vi "CAP1208 Example.vi"() -> ()   [LabVIEW 2020]
uses:
  <vilib>/MakerHub/LINX/Public/Utilities/Open Local.vi
  LINX I2C/LINX I2C.lvclass
  <vilib>/MakerHub/LINX/LMH-LINX.lvlib
  CAP1208/CAP1208.lvclass
panel:
  out "Sensor Input (CS1-CS8)":bool[](array[boolean])
  out "error out":errorcluster
  in  "Stop":bool
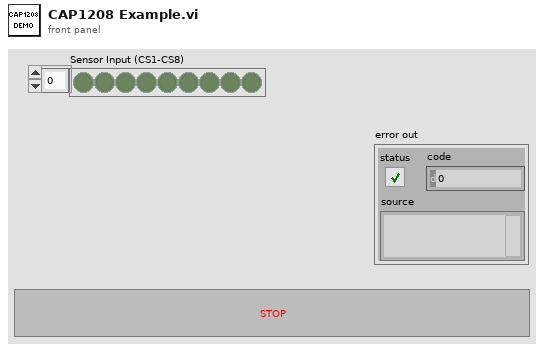
[diagram p1: front panel]
types:
  T1 = typedef "LMH-LINX.lvlib/LINX Ref.ctl" = cluster{"IO":T2, "Interface":T3, "LINX Device Config":T4}
  T2 = typedef "LMH-LINX.lvlib/Platform.ctl" = enum16{"Remote", "Local"}
  T3 = typedef "LMH-LINX.lvlib/Interface.ctl" = enum16{"Serial", "TCP"}
  T4 = typedef "LMH-LINX.lvlib/Device.lvlib/LINX Device Config.ctl" = cluster{"Interface":T3, "COM Port":refnum<visa-resource-name>, "TCP Configuration":T5, "Device Family":u8, "Device ID":u8, "Device Name":string, "TCP Ref":refnum<k5>, "Channels":T6}
  T5 = typedef "LMH-LINX.lvlib/Device.lvlib/TCP Config.ctl" = cluster{"IP Address":string, "Port":u16}
  T6 = typedef "LMH-LINX.lvlib/Channels.ctl" = cluster{"DI":u8[], "DO":u8[], "AI":u8[], "AO":u8[], "PWM":u8[], "QE":u8[], "UART":u8[], "I2C 2":u8[], "SPI":u8[], "CAN":u8[], "Servo":u8[], "AI Ref (V)":dbl, "AI Resolution (Bits)":u8, "AO Ref (V)":dbl, "AO Resolution (Bits)":u8}
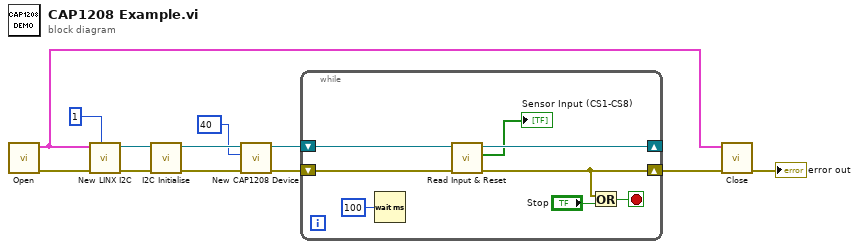
[diagram p0: block diagram]
diagram:
  n1 = call-poly <vilib>:"Open.vi"() -> ("Error Out"=w10:errorcluster, "LINX Resource"=w2:T1)  [unwired: 9 in, 1 out]
  n2 = call "New LINX I2C.vi"("LINX I2C Channel"=u8 1 ("I2C Channel"), "error in (no error)"=w10, "LINX Resource"=w2) -> ("error out"=w9:errorcluster, "LINX I2C out"=w11:refnum<class "LINX I2C.lvclass">)  [unwired: 7 in]
  n3 = call-dynamic "I2C Initialise.vi"("error in (no error)"=w9, "LINX I2C in"=w11) -> ("error out"=w8:errorcluster, "LINX I2C out"=w7:refnum<class "LINX I2C.lvclass">)  [unwired: 8 in]
  n4 = call "New CAP1208 Device.vi"("error in (no error)"=w8, "I2C Slave Address (0x28)"=u8 40, "I2C"=w7) -> ("error out"=w5:errorcluster, "CAP1208 out"=w4:refnum<class "CAP1208.lvclass">)  [unwired: 7 in]
  n5 = while {
    shift-right: [w15] -> _
    shift-left: w4 -> [w17]
    shift-right: [w14] -> w3
    shift-left: w5 -> [w16]
    stop <- w19 stop-if-true
    n6 = Wait (ms)(milliseconds to wait=u32 100) -> ()  [unwired: 1 out]
    n7 = call "Read Input & Reset.vi"("error in (no error)"=w16, "CAP1208 in"=w17) -> ("error out"=w14:errorcluster, "Sensor Input (CS1-CS8)"=→"Sensor Input (CS1-CS8)":bool[], "CAP1208 out"=w15:refnum<class "CAP1208.lvclass">)  [unwired: 6 in, 1 out]
    n8 = Or(x=w14, y="Stop") -> (x .or. y?=w19:bool)
  }
  n9 = call <vilib>:"Close.vi"("Error In"=w3, "LINX Resource"=w2) -> ("Error Out"=→"error out":errorcluster)  [unwired: 9 in]
